vi "copy IPF.vi"(8 "error in":errorcluster, 9 "APG Config":T1, 10 "Programs List":i32(listbox)) -> (0 "error out":errorcluster, 2 "New program name":string)   [LabVIEW 2013, in "Manipulate IPF.lvlib"]
uses:
  Manipulate IPF.lvlib
  Settings/type_def/APG Config.ctl
  Pack Data/type_def/file types.ctl
  <userlib>/_OpenG.lib/file/file.llb/Strip Path Extension - String__ogtk.vi
  <userlib>/_OpenG.lib/file/file.llb/Convert File Extension (String)__ogtk.vi
  Pack Data/Pack Files.lvlib
  Pack Data/type_def/command.ctl
  3013/code/a3Di.lvlib
  Settings/APG_settings.lvlib
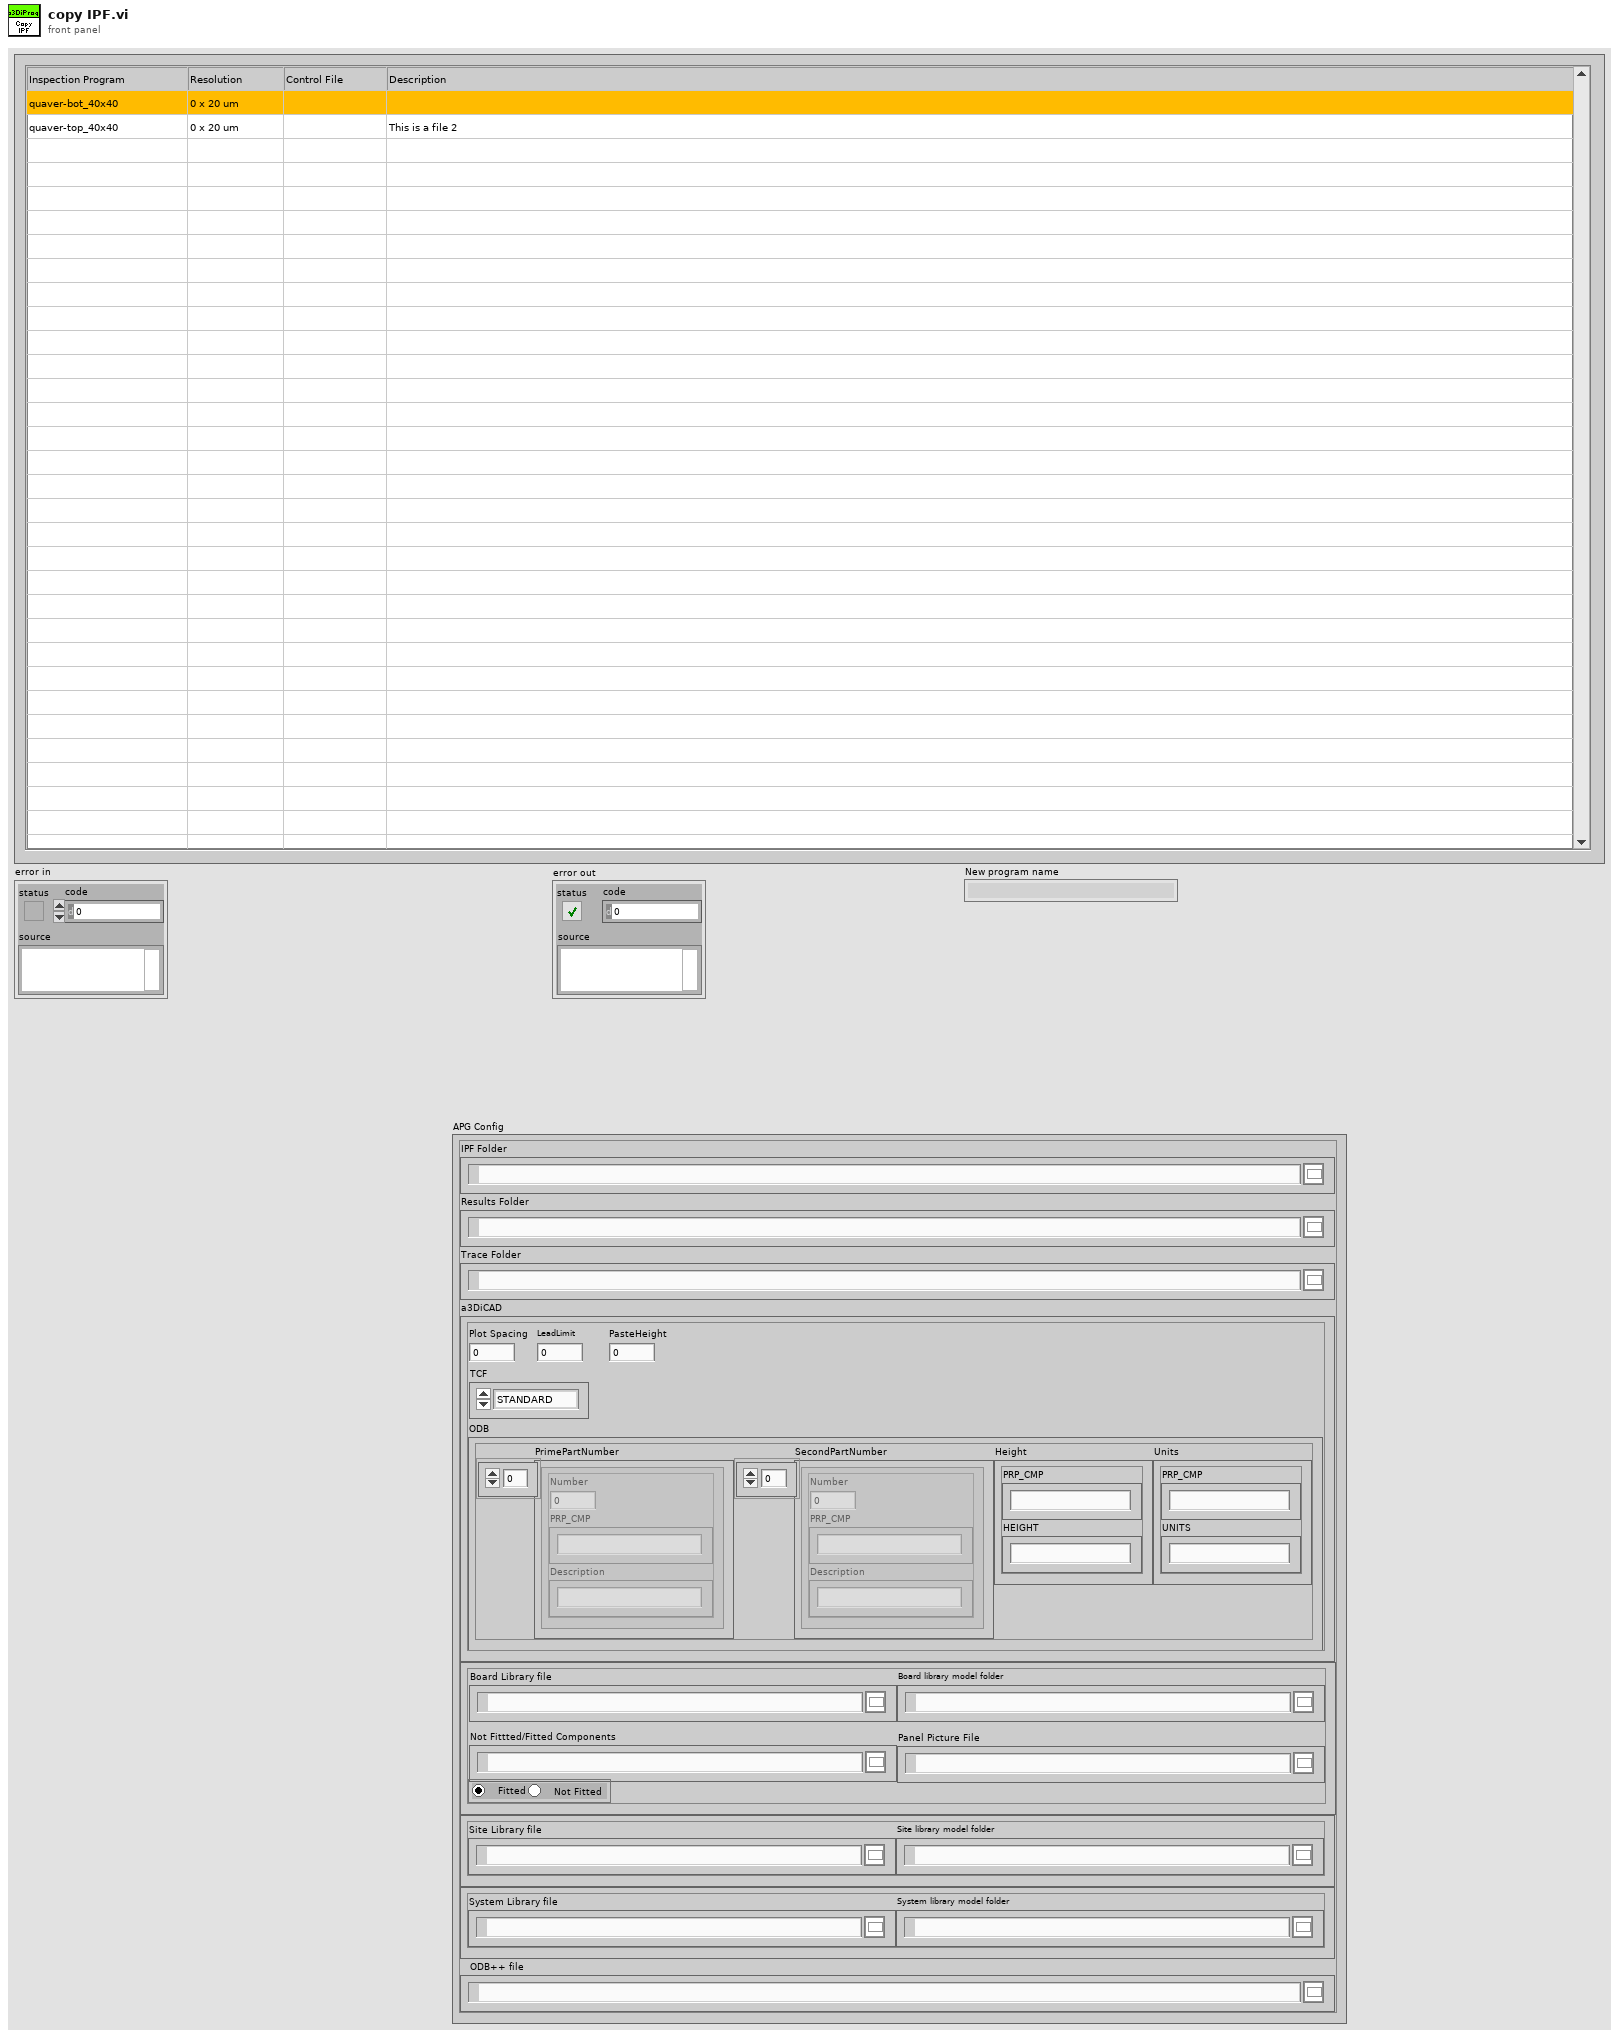
[diagram p1: front panel]
types:
  T1 = typedef "APG_settings.lvlib/APG Config.ctl" = cluster{"IPF Folder":path, "Results Folder":path, "Trace Folder":path, "a3DiCAD":cluster{"Plot Spacing":dbl, "TCF":enum16{"STANDARD", "PASTE", "LEAD"}, "LeadLimit":u32, "a3DiCADDebug":bool, "ODB":cluster{"PrimePartNumber":cluster{"Number":u32, "PRP_CMP":string, "Description":string}[], "SecondPartNumber":cluster{"Number":u32, "PRP_CMP":string, "Description":string}[], "Height":cluster{"PRP_CMP":string, "HEIGHT":string}, "Units":cluster{"PRP_CMP":string, "UNITS":string}}, "PasteHeight":dbl}, "a3DiCADcfg":path, "Board Library":cluster{"Board Library file":path, "Board library model folder":path, "Not Fittted/Fitted Components":path, "Panel Picture File":path, "Components":enum32{"Fitted", "Not Fitted "}}, "Site Library":cluster{"Site Library file":path, "Site library model folder":path}, "System Library":cluster{"System Library file":path, "System library model folder":path}, "ODB++ file":path}
  T2 = typedef "Pack Files.lvlib/file types.ctl" = enum16{"ODB", "TCF", "CAD Outline", "Config", "Inspection Prog", "a3Di-bin", "Results", "CAD Labels", "CAD Pads", "calScan_fid", "calScan_cal-tab", "PCB_SerialNumber", "CAD_Assembly", "Version", "Old Results", "CAD Picture", "Old TCF"}
  T3 = typedef "Pack Files.lvlib/command.ctl" = enum16{"Write", "Tar contents", "Read from Tar to File", "Delete", "Clean up Tar"}
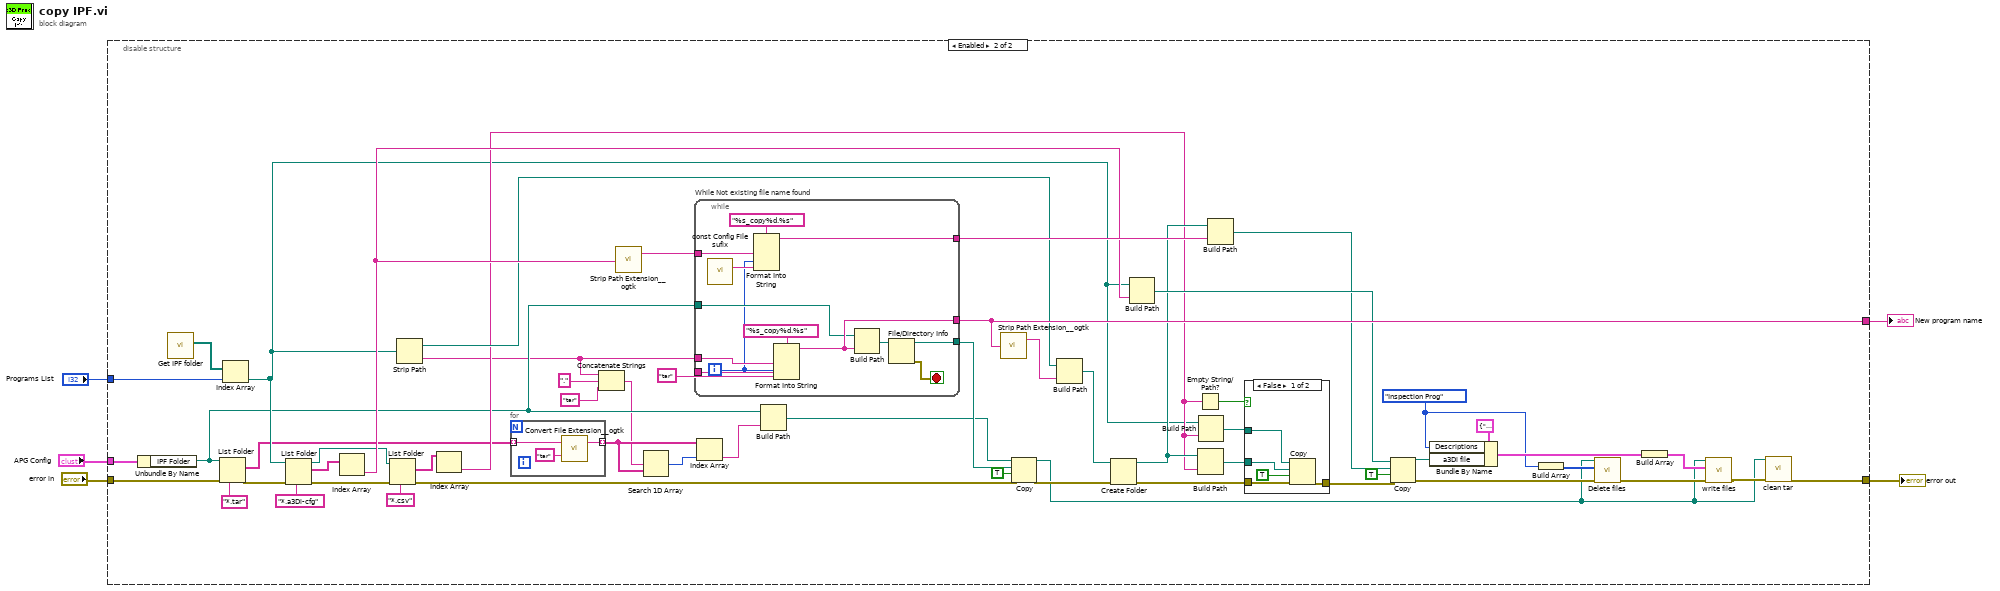
[diagram p0: block diagram]
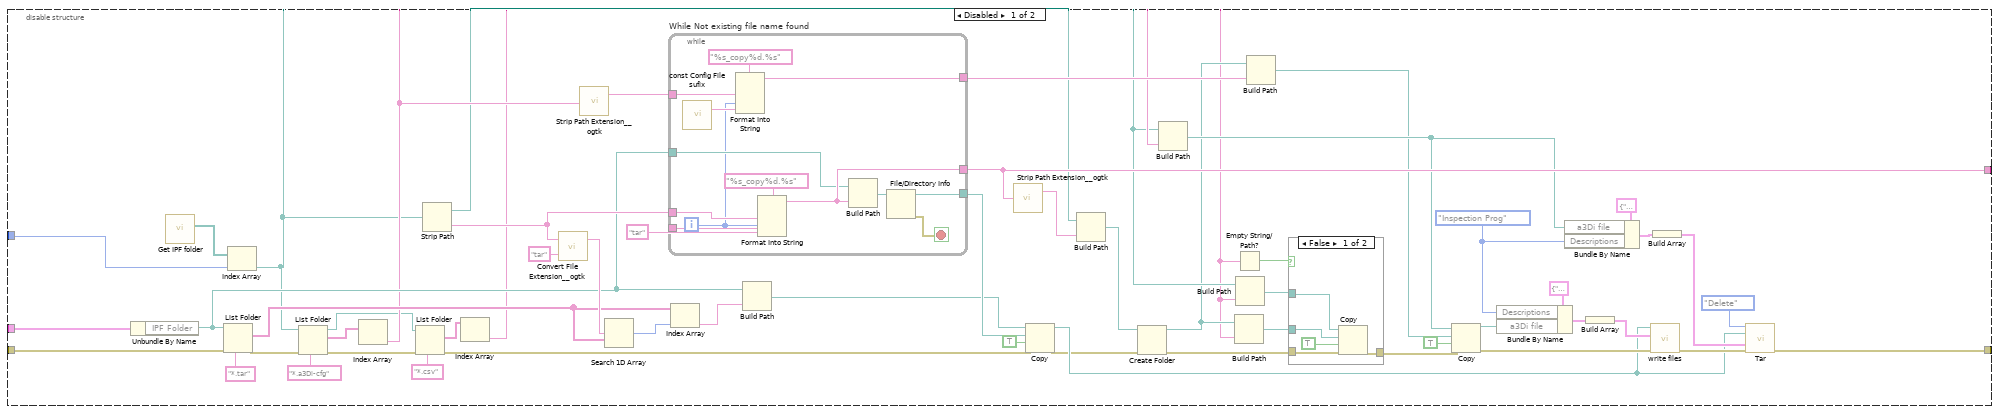
[diagram p2: hidden frame]
diagram:
  n1 = disable-structure shown="Enabled" {
    disable-tunnel: "error in" -> [w61 w136]
    disable-tunnel: [w60 w135] -> w4
    disable-tunnel: "Programs List" -> [w59 w134]
    disable-tunnel: "APG Config" -> [w58 w133]
    disable-tunnel: [w57 w92] -> w1
    frame Disabled {
      w39 = file_types."Inspection Prog" ("Descriptions")
      n2 = Unbundle By Name(w58) -> ("IPF Folder"=w37:path)
      n3 = call "Get IPF folder.vi"() -> ("IPF sub folders"=w56:path[])  [unwired: 6 in, 5 out]
      n4 = List Folder(path=w37, pattern="*.tar", error in=w61) -> (filenames=w34:string[], error out=w32:errorcluster)  [unwired: 1 in, 2 out]
      n5 = Index Array(array=w56, index=w59) -> (element=w13:path)
      n6 = List Folder(path=w13, pattern="*.a3Di-cfg", error in=w32) -> (path out=w6:path, filenames=w31:string[], error out=w19:errorcluster)  [unwired: 1 in, 1 out]
      n7 = Index Array(array=w31) -> (element=w26:string)  [unwired: 1 in]
      n8 = List Folder(path=w6, pattern="*.csv", error in=w19) -> (filenames=w16:string[], error out=w18:errorcluster)  [unwired: 1 in, 2 out]
      n9 = Strip Path(path=w13) -> (stripped path=w21:path, name=w48:string)
      n10 = Index Array(array=w16) -> (element=w9:string)  [unwired: 1 in]
      n11 = call-poly <userlib>:"Convert File Extension__ogtk.vi"("new ending (none)"="tar", "file name"=w48) -> ("new filename"=w49:string)  [unwired: 1 out]
      n12 = call-poly <userlib>:"Strip Path Extension__ogtk.vi"("path"=w26) -> ("root"=w30:string)  [unwired: 1 out]
      n13 = Search 1D Array(1D array=w34, element=w49) -> (index of element=w54:i32)  [unwired: 1 in]
      n14 = while "While Not existing file name found" {
        tunnel: "tar" -> [w77]
        tunnel: w48 -> [w78]
        tunnel: [w75] -> w60
        tunnel: [w74] -> w51
        tunnel: w37 -> [w73]
        tunnel: [w69] -> w36
        tunnel: w30 -> [w68]
        i -> [w70]
        stop <- w79 stop-if-true
        n15 = call "const Config File sufix.vi"() -> ("suffix"=w71:string)  [unwired: 14 in, 1 out]
        n16 = Format Into String(format string="%s_copy%d.%s", w68, w70, w71) -> (resulting string=w69:string)  [unwired: 2 in, 1 out]
        n17 = Format Into String(format string="%s_copy%d.%s", w78, w70, w77) -> (resulting string=w75:string)  [unwired: 2 in, 1 out]
        n18 = Build Path(base path=w73, name or relative path=w75) -> (appended path=w80:path)
        n19 = File/Directory Info(path=w80) -> (path out=w74:path, error out=w79:errorcluster)  [unwired: 1 in, 5 out]
      }
      n20 = Index Array(array=w34, index=w54) -> (element=w53:string)
      n21 = Build Path(base path=w37, name or relative path=w53) -> (appended path=w38:path)
      n22 = call-poly <userlib>:"Strip Path Extension__ogtk.vi"("path"=w60) -> ("root"=w22:string)  [unwired: 1 out]
      n23 = Copy(8:w18, 9:TRUE ("overwrite (F)"), 10:w51, 11:w38) -> (0:w23:errorcluster, 3:w27:path)  [unwired: 1 in, 1 out]
      n24 = Build Path(base path=w21, name or relative path=w22) -> (appended path=w20:path)
      n25 = Create Folder(path (use dialog)=w20, error in=w23) -> (created path=w11:path, error out=w15:errorcluster)  [unwired: 1 in, 1 out]
      n26 = Build Path(base path=w13, name or relative path=w26) -> (appended path=w25:path)
      n27 = Empty String/Path?(string/path=w9) -> (empty?=w8:bool)
      n28 = Build Path(base path=w11, name or relative path=w9) -> (appended path=w10:path)
      n29 = Build Path(base path=w13, name or relative path=w9) -> (appended path=w12:path)
      n30 = Build Path(base path=w11, name or relative path=w36) -> (appended path=w7:path)
      n31 = case shown="False" w8 {
        tunnel: w15 -> [w66 w67]
        tunnel: [w65 w67] -> w14
        tunnel: w12 -> [w64 _]
        tunnel: w10 -> [w63 _]
        frame False {
          n32 = Copy(8:w66, 9:TRUE ("overwrite (F)"), 10:w63, 11:w64) -> (0:w65:errorcluster)  [unwired: 1 in, 2 out]
        }
        frame True {
        }
      }
      n33 = Copy(8:w14, 9:TRUE ("overwrite (F)"), 10:w7, 11:w25) -> (0:w29:errorcluster, 3:w28:path)  [unwired: 1 in, 1 out]
      n34 = Bundle By Name(cluster=cluster{"Descriptions":T2, "a3Di file":path} {"Descriptions"=enum."ODB", "a3Di file"=path ""} ("Cluster"), "Descriptions"=w39, "a3Di file"=w28) -> (w41:cluster{"Descriptions":T2, "a3Di file":path})
      n35 = Bundle By Name(cluster=cluster{"Descriptions":T2, "a3Di file":path} {"Descriptions"=enum."ODB", "a3Di file"=path ""} ("Cluster"), "a3Di file"=w25, "Descriptions"=w39) -> (w46:cluster{"Descriptions":T2, "a3Di file":path})
      n36 = Build Array(w41) -> (w40:cluster{"Descriptions":T2, "a3Di file":path}[])
      n37 = call "write files.vi"("error in (no error)"=w29, "Files to be zipped"=w40, "a3Di  tar file"=w27) -> ("error out"=w47:errorcluster)  [unwired: 7 in, 1 out]
      n38 = Build Array(w46) -> (w43:cluster{"Descriptions":T2, "a3Di file":path}[])
      n39 = call "Tar.vi"("Command"=command."Delete", "a3Di  tar file"=w27, "a3Di Files"=w43, "error in (no error)"=w47) -> ("error out"=w57:errorcluster)  [unwired: 8 in, 3 out]
    }
    frame Enabled {
      w95 = file_types."Inspection Prog" ("Descriptions")
      n40 = Unbundle By Name(w133) -> ("IPF Folder"=w87:path)
      n41 = call "Get IPF folder.vi"() -> ("IPF sub folders"=w132:path[])  [unwired: 6 in, 5 out]
      n42 = List Folder(path=w87, pattern="*.tar", error in=w136) -> (filenames=w86:string[], error out=w121:errorcluster)  [unwired: 1 in, 2 out]
      n43 = Index Array(array=w132, index=w134) -> (element=w90:path)
      n44 = List Folder(path=w90, pattern="*.a3Di-cfg", error in=w121) -> (path out=w98:path, filenames=w120:string[], error out=w110:errorcluster)  [unwired: 1 in, 1 out]
      n45 = Index Array(array=w120) -> (element=w117:string)  [unwired: 1 in]
      n46 = List Folder(path=w98, pattern="*.csv", error in=w110) -> (filenames=w107:string[], error out=w109:errorcluster)  [unwired: 1 in, 2 out]
      n47 = Strip Path(path=w90) -> (stripped path=w112:path, name=w82:string)
      n48 = Index Array(array=w107) -> (element=w101:string)  [unwired: 1 in]
      n49 = for {
        tunnel: [w139] -> w85 mode=indexing
        tunnel: w86 -> [w138] mode=indexing
        n50 = call-poly <userlib>:"Convert File Extension__ogtk.vi"("new ending (none)"="tar", "file name"=w138) -> ("new filename"=w139:string)  [unwired: 1 out]
      }
      n51 = Concatenate Strings(w82, "." ("string"), "tar" ("new ending (none)")) -> (w81:string)
      n52 = call-poly <userlib>:"Strip Path Extension__ogtk.vi"("path"=w117) -> ("root"=w119:string)  [unwired: 1 out]
      n53 = Search 1D Array(1D array=w85, element=w81) -> (index of element=w130:i32)  [unwired: 1 in]
      n54 = while "While Not existing file name found" {
        tunnel: "tar" -> [w155]
        tunnel: w82 -> [w156]
        tunnel: [w153] -> w135
        tunnel: [w152] -> w127
        tunnel: w87 -> [w151]
        tunnel: [w147] -> w122
        tunnel: w119 -> [w146]
        i -> [w148]
        stop <- w157 stop-if-true
        n55 = call "const Config File sufix.vi"() -> ("suffix"=w149:string)  [unwired: 14 in, 1 out]
        n56 = Format Into String(format string="%s_copy%d.%s", w146, w148, w149) -> (resulting string=w147:string)  [unwired: 2 in, 1 out]
        n57 = Format Into String(format string="%s_copy%d.%s", w156, w148, w155) -> (resulting string=w153:string)  [unwired: 2 in, 1 out]
        n58 = Build Path(base path=w151, name or relative path=w153) -> (appended path=w158:path)
        n59 = File/Directory Info(path=w158) -> (path out=w152:path, error out=w157:errorcluster)  [unwired: 1 in, 5 out]
      }
      n60 = Index Array(array=w85, index=w130) -> (element=w129:string)
      n61 = Build Path(base path=w87, name or relative path=w129) -> (appended path=w123:path)
      n62 = call-poly <userlib>:"Strip Path Extension__ogtk.vi"("path"=w135) -> ("root"=w113:string)  [unwired: 1 out]
      n63 = Copy(8:w109, 9:TRUE ("overwrite (F)"), 10:w127, 11:w123) -> (0:w114:errorcluster, 3:w91:path)  [unwired: 1 in, 1 out]
      n64 = Build Path(base path=w112, name or relative path=w113) -> (appended path=w111:path)
      n65 = Create Folder(path (use dialog)=w111, error in=w114) -> (created path=w103:path, error out=w106:errorcluster)  [unwired: 1 in, 1 out]
      n66 = Build Path(base path=w90, name or relative path=w117) -> (appended path=w116:path)
      n67 = Empty String/Path?(string/path=w101) -> (empty?=w100:bool)
      n68 = Build Path(base path=w103, name or relative path=w101) -> (appended path=w102:path)
      n69 = Build Path(base path=w90, name or relative path=w101) -> (appended path=w104:path)
      n70 = Build Path(base path=w103, name or relative path=w122) -> (appended path=w99:path)
      n71 = case shown="False" w100 {
        tunnel: w106 -> [w144 w145]
        tunnel: [w143 w145] -> w105
        tunnel: w104 -> [w142 _]
        tunnel: w102 -> [w141 _]
        frame False {
          n72 = Copy(8:w144, 9:TRUE ("overwrite (F)"), 10:w141, 11:w142) -> (0:w143:errorcluster)  [unwired: 1 in, 2 out]
        }
        frame True {
        }
      }
      n73 = Copy(8:w105, 9:TRUE ("overwrite (F)"), 10:w99, 11:w116) -> (0:w97:errorcluster, 3:w118:path)  [unwired: 1 in, 1 out]
      n74 = Bundle By Name(cluster=cluster{"Descriptions":T2, "a3Di file":path} {"Descriptions"=enum."ODB", "a3Di file"=path ""} ("Cluster"), "Descriptions"=w95, "a3Di file"=w118) -> (w125:cluster{"Descriptions":T2, "a3Di file":path})
      n75 = Build Array(w95) -> (w94:T2[])
      n76 = call "Delete files.vi"("error in (no error)"=w97, "File type[]"=w94, "a3Di  tar file"=w91) -> ("error out"=w96:errorcluster)  [unwired: 8 in]
      n77 = Build Array(w125) -> (w124:cluster{"Descriptions":T2, "a3Di file":path}[])
      n78 = call "write files.vi"("error in (no error)"=w96, "Files to be zipped"=w124, "a3Di  tar file"=w91) -> ("error out"=w93:errorcluster)  [unwired: 7 in, 1 out]
      n79 = call "clean tar.vi"("tar file"=w91, "error in (no error)"=w93) -> ("error out"=w92:errorcluster)  [unwired: 13 in]
    }
  }
  "error out" <- w1
  "New program name" <- w4
